vi "Read v_y.vi"(8 "error in (no error)":errorcluster, 11 "Vector in":refnum<class "Vector.lvclass">) -> (0 "error out":errorcluster, 2 "P_x":refnum<class "Rational Number.lvclass">, 3 "Vector out":refnum<class "Vector.lvclass">)   [LabVIEW 2021, in "Vector.lvclass"]
uses:
  Vector.lvclass
  Vector.lvclass/Vector.ctl
  High Res Arithmetic/Rational Number.lvclass
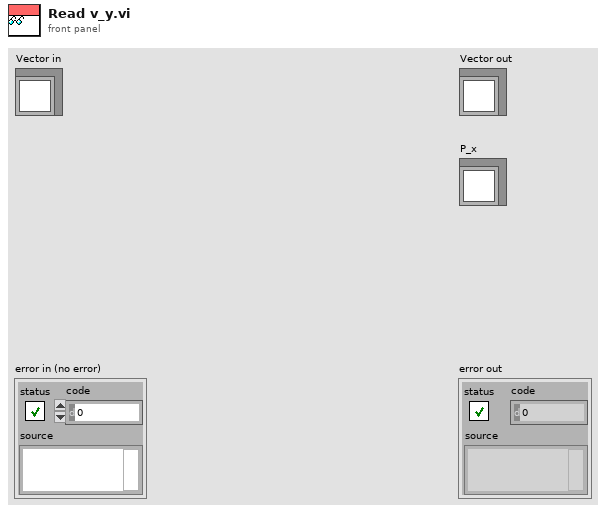
[diagram p1: front panel]
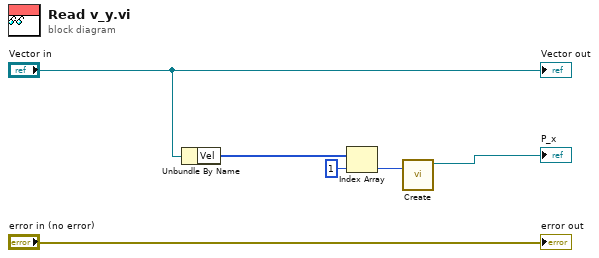
[diagram p0: block diagram]
diagram:
  n1 = Unbundle By Name("Vector in") -> ("Vel"=w3:i64[])
  n2 = Index Array(array=w3, index=1) -> (element=w2:i64)
  n3 = call "Create.vi"("Numerator"=w2) -> ("Hi Res Arithm Test"=→"P_x":refnum<class "Rational Number.lvclass">)  [unwired: 9 in, 1 out]
  "error out" <- "error in (no error)"
  "Vector out" <- "Vector in"
